vi "InverseModelOptForm.vi"() -> ()   [LabVIEW 2012]
panel:
  in  "Default":bool
  in  "Cancel Button":bool
  in  "OK Button":bool
  in  "AccValue":dbl caption="Merit value for \"acceptable\" fit:"
  in  "GoodValue":dbl caption="Merit value for \"good\" fit:"
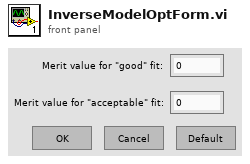
[diagram p1: front panel]
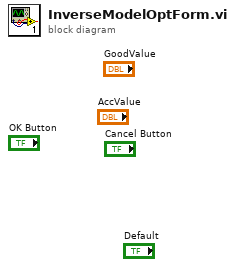
[diagram p0: block diagram]
diagram:
